vi "Reaper Singleton.vi"(9 "Write? (F)":bool, 11 "Reaper In":refnum<class "Reaper.lvclass">) -> (3 "Reaper Out":refnum<class "Reaper.lvclass">)   [LabVIEW 2015, in "Reaper.lvclass"]
uses:
  Reaper.lvclass
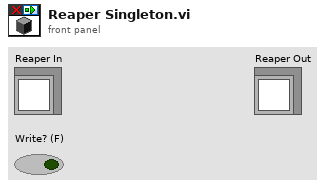
[diagram p1: front panel]
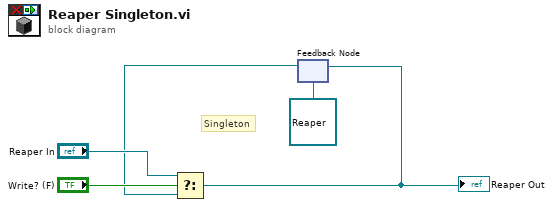
[diagram p0: block diagram]
diagram:
  # "Singleton"
  n1 = feedback #1(refnum<class "Reaper.lvclass"> refnum ("Reaper.lvclass")) -> (w2:refnum<class "Reaper.lvclass">)
  n2 = Select(t="Reaper In", s="Write? (F)", f=w2) -> (s? t:f=w1:refnum<class "Reaper.lvclass">)
  "Reaper Out" <- w1
  n3 = feedback-in #1(w1) -> ()
